vi "Datasheet Find Channel by Name.vi"(10 "Channel Name":string, 11 "Channel Data":T1[](array[typedef])) -> (2 "Waveform":dbl[](array[numeric]), 3 "index of element":i32)   [LabVIEW 2011]
uses:
  TDMS/TDMS Channel (Sxx).ctl
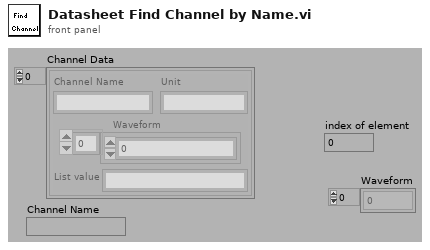
[diagram p1: front panel]
types:
  T1 = typedef "TDMS Channel (Sxx).ctl" = cluster{"Channel Name":string, "Waveform":dbl[], "Unit":string, "List value":string}
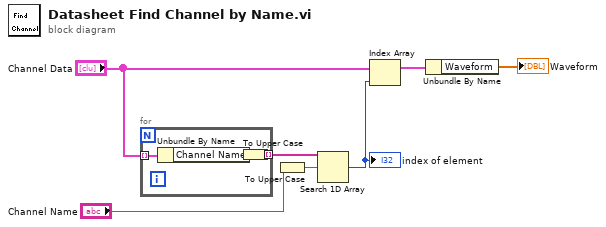
[diagram p0: block diagram]
diagram:
  n1 = for {
    tunnel: "Channel Data" -> [w10] mode=indexing
    tunnel: [w8] -> w5 mode=indexing
    n2 = Unbundle By Name(w10) -> ("Channel Name"=w9:string)
    n3 = To Upper Case(1:w9) -> (0:w8:string)
  }
  n4 = To Upper Case(1:"Channel Name") -> (0:w7:string)
  n5 = Search 1D Array(1D array=w5, element=w7) -> (index of element=w3:i32)  [unwired: 1 out]
  "index of element" <- w3
  n6 = Index Array(array="Channel Data", index=w3) -> (element=w2:T1)
  n7 = Unbundle By Name(w2) -> ("Waveform"=→"Waveform":dbl[])
